vi "launcher.vi"(8 "error in":errorcluster, 11 "communicator in":refnum<class "communicator.lvclass">) -> (0 "error out":errorcluster)   [LabVIEW 2015, in "communicator.lvclass"]
uses:
  communicator.lvclass
  static background worker.vi
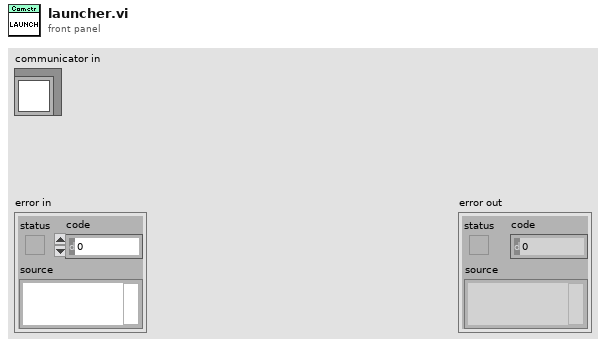
[diagram p1: front panel]
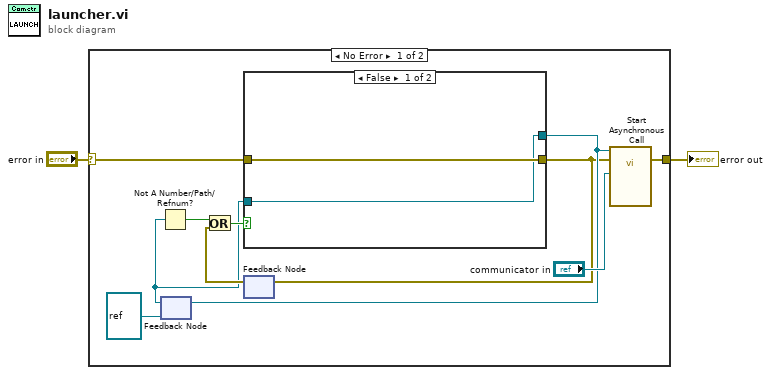
[diagram p0: block diagram]
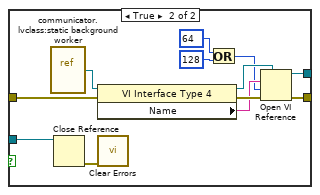
[diagram p2: hidden frame]
diagram:
  n1 = case shown="No Error" "error in" {
    selector: "error in" -> [w12 w27]
    tunnel: [w10 w27] -> w1
    frame No Error {
      n2 = feedback #1(refnum<vi> refnum) -> (w3:refnum<vi>)
      n3 = Not A Number/Path/Refnum?(number/path/refnum=w3) -> (NaN/Path/Refnum?=w5:bool)
      n4 = feedback #2() -> (w6:errorcluster)  [unwired: 1 in]
      n5 = Or(x=w5, y=w6) -> (x .or. y?=w4:bool)
      n6 = case shown="False" w4 {
        tunnel: w12 -> [w14 w19]
        tunnel: [w13 w18] -> w9
        tunnel: [w14 w17] -> w7
        tunnel: w3 -> [w13 w16]
        frame False {
        }
        frame True {
          n7 = vi-ref "communicator.lvclass:static background worker.vi"() -> (w22:refnum<vi>)
          n8 = Close Reference(reference=w16) -> (error out=w15:errorcluster)  [unwired: 1 in]
          n9 = property class="VI Interface Type 4"(reference=w22, error in=w19) -> (reference out=w24:refnum<vi>, error out=w26:errorcluster, "Name"=w25:string)
          n10 = call <vilib>:"Clear Errors.vi"("error in (no error)"=w15) -> ()  [unwired: 5 in, 2 out]
          n11 = Or(x=64 ("options"), y=128 ("options")) -> (x .or. y?=w23:i32)
          n12 = Open VI Reference(type specifier VI Refnum (for type only)=w24, vi path=w25, options=w23, error in (no error)=w26) -> (vi reference=w18:refnum<vi>, error out=w17:errorcluster)  [unwired: 2 in]
        }
      }
      n13 = feedback-in #1(w9) -> ()
      n14 = feedback-in #2(w7) -> ()
      n15 = call-by-ref "Start Asynchronous Call"(reference=w9, error in=w7, "communicator in"="communicator in") -> (error out=w10:errorcluster)  [unwired: 11 in, 1 out]
    }
    frame Error {
    }
  }
  "error out" <- w1
